vi "Init.vi"(8 "error in":errorcluster, 11 "DAQmx Base CFG in":refnum<class "DAQmx Base CFG.lvclass">) -> (0 "error out":errorcluster, 3 "DAQmx Base CFG out":refnum<class "DAQmx Base CFG.lvclass">)   [LabVIEW 2023, in "DAQmx Base CFG.lvclass"]
uses:
  DAQmx Base CFG.lvclass
  DAQmx Base CFG.lvclass/DAQmx Base CFG.ctl
  <vilib>/Utility/error.llb/Error Cluster From Error Code.vi
  CFG Target/CFG Target.lvclass
  <vilib>/ErrorRing/Error Ring.xnode
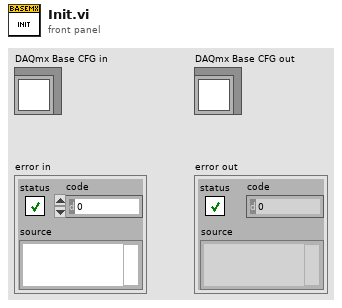
[diagram p1: front panel]
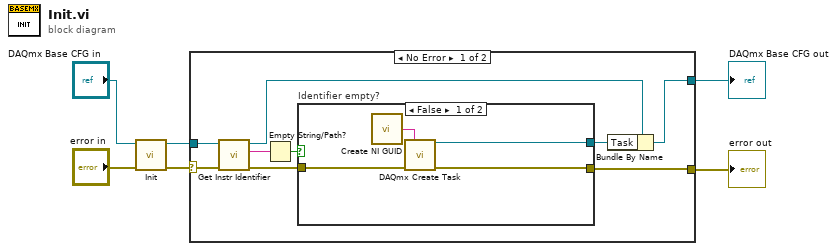
[diagram p0: block diagram]
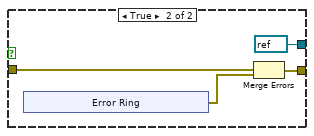
[diagram p2: hidden frame]
diagram:
  n1 = call-parent "Init.vi"("error in (no error)"="error in", "CFG Base in"="DAQmx Base CFG in") -> ("error out"=w3:errorcluster, "CFG Base out"=w1:refnum<class "DAQmx Base CFG.lvclass">)  [unwired: 8 in]
  n2 = case shown="No Error" w3 {
    selector: w3 -> [w15 w29]
    tunnel: w1 -> [w14 w30]
    tunnel: [w8 w30] -> w5
    tunnel: [w10 w29] -> w4
    frame No Error {
      n3 = call-dynamic "Get Instr Identifier.vi"("error in (no error)"=w15, "Configuration Base in"=w14) -> ("error out"=w11:errorcluster, "Instr Ident"=w13:string, "Configuration Base out"=w9:refnum<class "DAQmx Base CFG.lvclass">)  [unwired: 7 in]
      n4 = Empty String/Path?(string/path=w13) -> (empty?=w12:bool)
      n5 = case "Identifier empty?" shown="False" w12 {
        tunnel: w11 -> [w19 w23]
        tunnel: [w18 w22] -> w10
        tunnel: [w16 refnum<k21> refnum ("task out")] -> w7
        frame False {
          n6 = call <vilib>:"Create NI GUID.vi"() -> ("NI GUID"=w17:string)
          n7 = call <vilib>:"DAQmx Create Task.vi"("new task name"=w17, "error in"=w19) -> ("task out"=w16:refnum<k21>, "error out"=w18:errorcluster)  [unwired: 12 in]
        }
        frame True {
          n8 = xnode "Error Ring"() -> ("error out"=w21:errorcluster)
          n9 = Merge Errors(w23, w21) -> (w22:errorcluster)
        }
      }
      n10 = Bundle By Name(cluster=w9, "Task"=w7) -> (w8:refnum<class "DAQmx Base CFG.lvclass">)
    }
    frame Error {
    }
  }
  "error out" <- w4
  "DAQmx Base CFG out" <- w5
